vi "Sort.vi"(7 "升降序":enum16{"升序", "降序"}(ring), 8 "错误输入":errorcluster, 10 "列索引":i32, 11 "Mlistbox Ref":refnum<vi>) -> (0 "错误输出":errorcluster, 3 "Mlistbox Ref Dup":refnum<vi>)   [LabVIEW 2012, in "Mlistbox Tools.lvlib"]
uses:
  Mlistbox Tools.lvlib
  ListBox/Custom Type/Read and Write Mode.ctl
  Property/Set and Get ItemNames.vi
  ListBox/Listbox Tool.lvlib
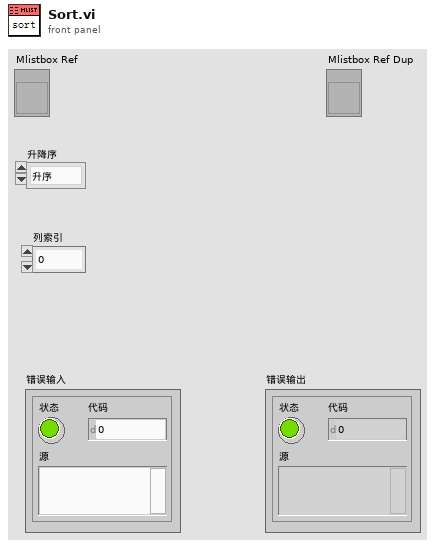
[diagram p1: front panel]
types:
  T1 = typedef "Listbox Tool.lvlib/Read and Write Mode.ctl" = enum16{"Read", "Write"}
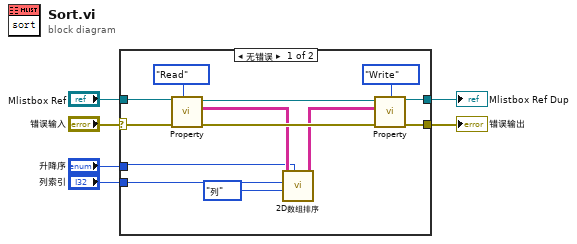
[diagram p0: block diagram]
diagram:
  n1 = case shown="无错误" "错误输入" {
    selector: "错误输入" -> [w16 w21]
    tunnel: [w14 w21] -> w5
    tunnel: "Mlistbox Ref" -> [w19 w20]
    tunnel: [w15 w20] -> w3
    tunnel: "升降序" -> [w9 _]
    tunnel: "列索引" -> [w7 _]
    frame No Error {
      n2 = call-poly "Property.vi"("Mode"=Read_and_Write_Mode."Read", "错误输入"=w16, "Mlistbox Ref"=w19) -> ("错误输出"=w12:errorcluster, "ItemNames Out"=w11:string[][], "Mlistbox Ref Dup"=w13:refnum<vi>)  [unwired: 6 in]
      n3 = call-poly "2D数组排序.vi"("升降序"=w9, "选择行列"=enum16{"行", "列"}."列", "行/列索引"=w7, "输入数组"=w11) -> ("排序后数组"=w10:string[][])  [unwired: 5 in, 2 out]
      n4 = call-poly "Property.vi"("Mode"=Read_and_Write_Mode."Write", "错误输入"=w12, "ItemNames In"=w10, "Mlistbox Ref"=w13) -> ("错误输出"=w14:errorcluster, "Mlistbox Ref Dup"=w15:refnum<vi>)  [unwired: 5 in, 1 out]
    }
    frame Error {
    }
  }
  "Mlistbox Ref Dup" <- w3
  "错误输出" <- w5
